vi "First1.vi"() -> ()   [LabVIEW 2020]
uses:
  First1Second1glb.vi
panel:
  in  "stop":bool
  out "Waveform Chart":dbl(graph)
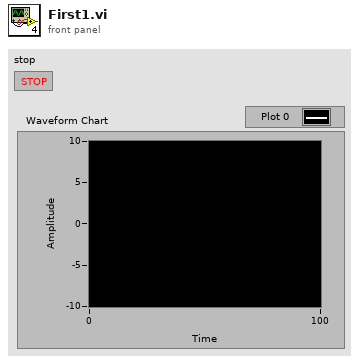
[diagram p1: front panel]
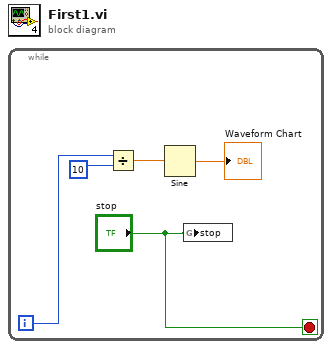
[diagram p0: block diagram]
diagram:
  n1 = while {
    i -> [w4]
    stop <- "stop" stop-if-true
    n2 = Divide(x=w4, y=10) -> (x/y=w3:dbl)
    n3 = Sine(x=w3) -> (sin(x)=→"Waveform Chart":dbl)
    n4 = global write "First1Second1glb.vi" "stop"("stop") -> ()
  }
